vi "Initialize Sessions Impl.vi"(6 "initialize and close session behavior":T1, 7 "require single session":bool, 8 "error in":errorcluster, 10 "instrument":refnum<class "ISession Factory.lvclass">, 11 "session reservation in":refnum<class "Session Reservation.lvclass">) -> (0 "error out":errorcluster, 1 "channel lists":string[](array[string]), 2 "sessions":variant[](array[variant]), 3 "session reservation out":refnum<class "Session Reservation.lvclass">, 4 "location unique id":u64, 5 "retry":bool)   [LabVIEW 2020, in "Measurement Plugin Session Management V1.lvlib" / "Session Reservation.lvclass"]
uses:
  Session Reservation.lvclass
  Sessions/Instrument Sessions/ISession Factory/ISession Factory.lvclass
  Initialize and Close Session Behavior.ctl
  Session Reservation.lvclass/Session Reservation.ctl
  Sessions/Instrument Sessions/ISession Factory/Session Initialization Parameters.ctl
  Measurement Plugin Measurement Server/Helpers/Error Strings Global Internal.vi
  Connection Map/Connection Map.lvclass
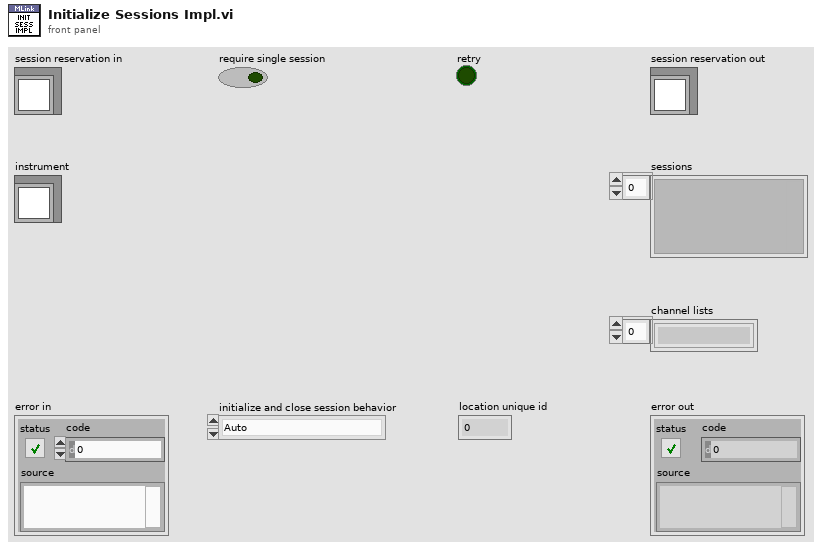
[diagram p1: front panel]
types:
  T1 = typedef "Measurement Plugin Session Management V1.lvlib/Session Reservation.lvclass/Initialize and Close Session Behavior.ctl" = enum16{"Auto", "Initialize and Close", "Attach and Detach", "Initialize and Detach", "Attach and Close"}
  T2 = typedef "Instrument Sessions.lvlib/ISession Factory.lvclass/Session Initialization Parameters.ctl" = cluster{"resource name":string, "session name":string}
  T3 = typedef "Measurement Plugin Session Management V1.lvlib/Session Reservation.lvclass/Data.ctl" = cluster{"session and driver infos":T4[], "pin or relay names":string[], "connection map":refnum<class "Connection Map.lvclass">, "pin map context":T9, "reservation observer":refnum<class "IReservation Observer.lvclass">, "dvr valid":bool, "group mappings":T10}
  T4 = typedef "Measurement Plugin Session Management V1.lvlib/Session Reservation.lvclass/Session and Driver Info.ctl" = cluster{"session info":T5, "session":variant, "session factory":refnum<class "ISession Factory.lvclass">, "initialize and close session behavior":T8}
  T5 = typedef "MeasurementLink Session Management Client.lvlib/ni_measurementlink_sessionmanagement_v1_SessionInformation.ctl" = cluster{"session":T6, "resource_name":string, "channel_list":string, "instrument_type_id":string, "session_exists":bool, "channel_mappings":T7[]}
  T6 = typedef "MeasurementLink Session Management Client.lvlib/nidevice_grpc_Session.ctl" = cluster{"name":string}
  T7 = typedef "MeasurementLink Session Management Client.lvlib/ni_measurementlink_sessionmanagement_v1_ChannelMapping.ctl" = cluster{"pin_or_relay_name":string, "site":i32, "channel":string, "multiplexer_resource_name":string, "multiplexer_route":string}
  T8 = typedef "Instrument Sessions.lvlib/ISession Factory.lvclass/Initialize and Close Session Behavior.ctl" = enum16{"Initialize and Close", "Attach and Detach", "Initialize and Detach", "Attach and Close"}
  T9 = typedef "MeasurementLink Session Management Client.lvlib/ni_measurementlink_PinMapContext.ctl" = cluster{"pin_map_id":string, "sites":i32[]}
  T10 = typedef "Measurement Plugin Session Management V1.lvlib/Session Reservation.lvclass/Group Mapping.ctl" = map{string, string[]}
  T11 = typedef "Instrument Sessions.lvlib/ISession Factory.lvclass/Remote Connection Options.ctl" = cluster{"session name":string, "address":string, "port":u32}
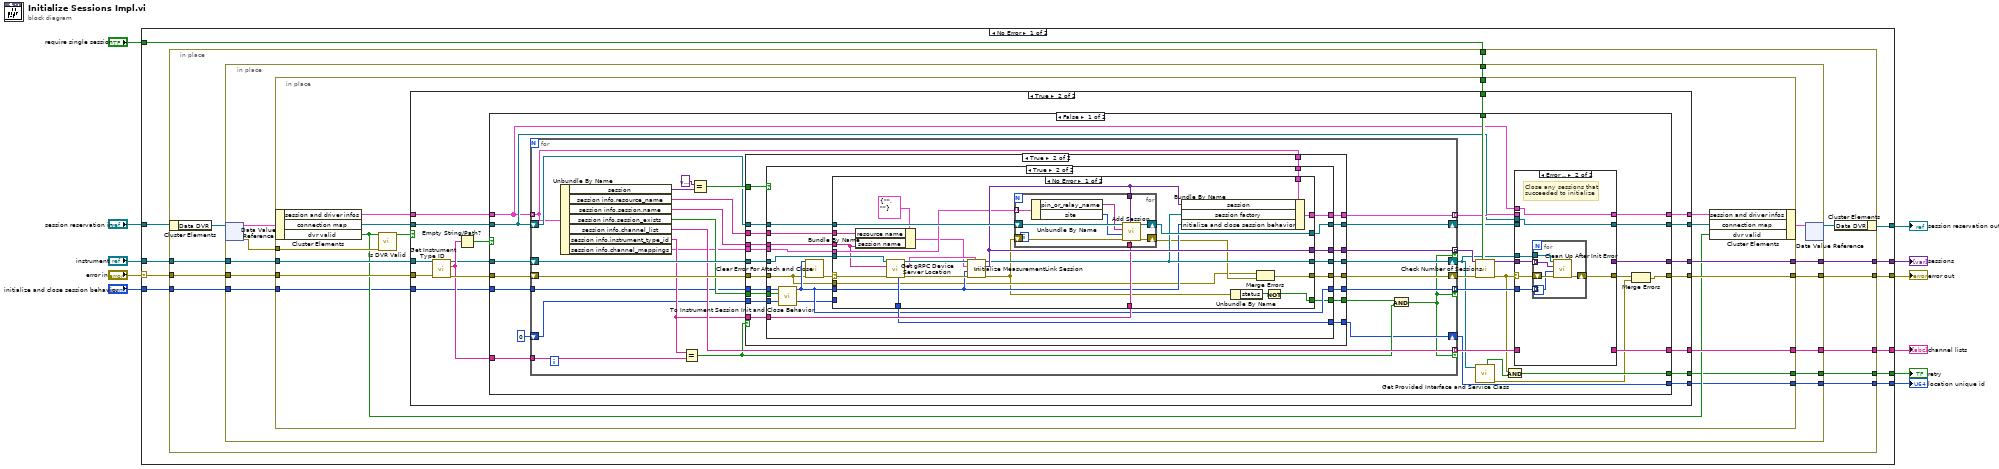
[diagram p0: block diagram]
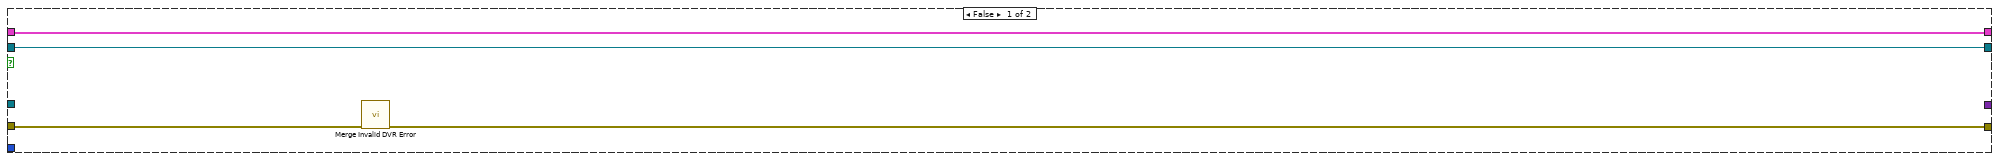
[diagram p2: hidden frame]
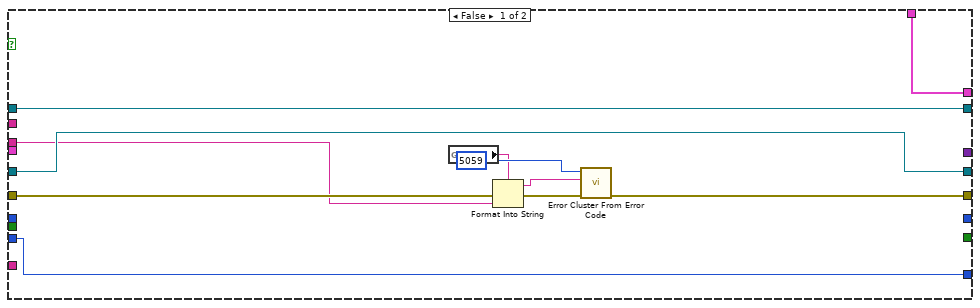
[diagram p5: hidden frame]
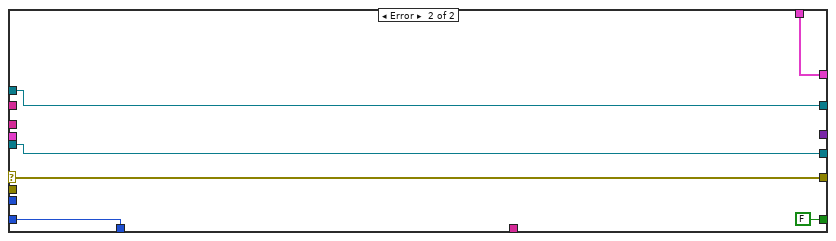
[diagram p6: hidden frame]
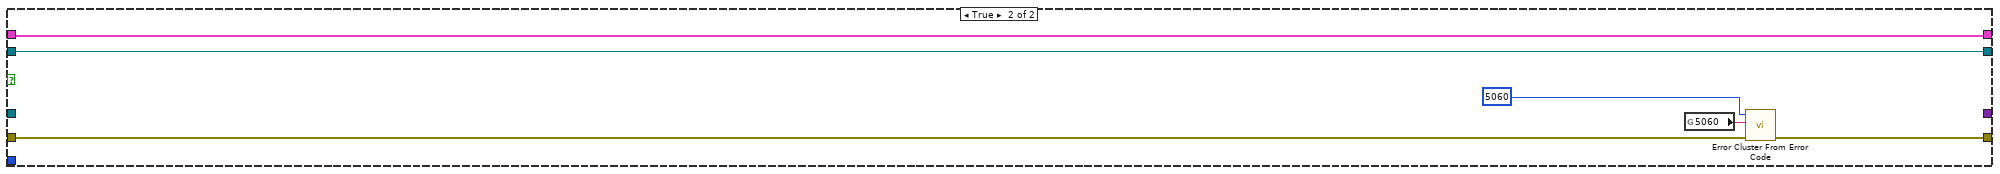
[diagram p7: hidden frame]
diagram:
  n1 = case shown="No Error" "error in" {
    selector: "error in" -> [w19 w256]
    tunnel: "session reservation in" -> [w16 w255]
    tunnel: "instrument" -> [w18 _]
    tunnel: [w22 _] -> w9
    tunnel: [w21 w256] -> w8
    tunnel: [w20 _] -> w7
    tunnel: [w15 w255] -> w4
    tunnel: "require single session" -> [w17 _]
    tunnel: "initialize and close session behavior" -> [w14 _]
    tunnel: [w13 _] -> w2
    tunnel: [w12 _] -> w1
    frame No Error {
      n2 = in-place {
        in-place-border: [w33] -> w22
        in-place-border: [w32] -> w21
        in-place-border: [w31] -> w20
        in-place-border: w19 -> [w30]
        in-place-border: w18 -> [w29]
        in-place-border: w17 -> [w28]
        in-place-border: w14 -> [w25]
        in-place-border: [w24] -> w13
        in-place-border: [w23] -> w12
        n3 = in-place-cluster #1(w16) -> ("Data DVR"=w27:refnum<data-value>)
        n4 = in-place {
          in-place-border: [w45] -> w33
          in-place-border: [w44] -> w32
          in-place-border: [w43] -> w31
          in-place-border: w30 -> [w42]
          in-place-border: w29 -> [w41]
          in-place-border: w28 -> [w40]
          in-place-border: w25 -> [w36]
          in-place-border: [w35] -> w24
          in-place-border: [w34] -> w23
          n5 = in-place-dvr #2(w27) -> (w39:T3, w38:errorcluster)
          n6 = in-place {
            in-place-border: [w61] -> w45
            in-place-border: [w60] -> w44
            in-place-border: [w59] -> w43
            in-place-border: w42 -> [w51]
            in-place-border: w41 -> [w50]
            in-place-border: w40 -> [w58]
            in-place-border: w38 -> [w54]
            in-place-border: w36 -> [w48]
            in-place-border: [w47] -> w35
            in-place-border: [w46] -> w34
            n7 = in-place-cluster #3(w39) -> ("session and driver infos"=w57:T4[], "connection map"=w56:refnum<class "Connection Map.lvclass">, "dvr valid"=w49:bool)
            n8 = call "Is DVR Valid.vi"("dvr error in"=w54, "dvr valid in"=w49) -> ("dvr valid out"=w53:bool)  [unwired: 9 in]
            n9 = case shown="True" w53 {
              tunnel: [_ w82] -> w61
              tunnel: [w62 w81] -> w60
              tunnel: [_ w80] -> w59
              tunnel: w58 -> [_ w79]
              tunnel: [w64 w78] -> w52
              tunnel: w57 -> [w64 w77]
              tunnel: w56 -> [w65 w76]
              tunnel: [w65 w75] -> w55
              tunnel: w51 -> [w63 w74]
              tunnel: w50 -> [_ w73]
              tunnel: w48 -> [_ w68]
              tunnel: [_ w67] -> w47
              tunnel: [_ w66] -> w46
              frame False {
                n10 = call "Merge Invalid DVR Error.vi"("error in"=w63) -> ("error out"=w62:errorcluster)  [unwired: 10 in]
              }
              frame True {
                n11 = call-dynamic "Get Instrument Type ID.vi"("error in"=w74, "session factory in"=w73) -> ("error out"=w72:errorcluster, "instrument type id"=w71:string, "session factory out"=w70:refnum<class "ISession Factory.lvclass">)  [unwired: 7 in]
                n12 = Empty String/Path?(string/path=w71) -> (empty?=w69:bool)
                n13 = case shown="False" w69 {
                  tunnel: w77 -> [w93 w254]
                  tunnel: [w109 _] -> w82
                  tunnel: [w85 w251] -> w81
                  tunnel: [w107 _] -> w80
                  tunnel: [w95 w254] -> w78
                  tunnel: w71 -> [w106 _]
                  tunnel: w70 -> [w105 _]
                  tunnel: w72 -> [w104 w250]
                  tunnel: w79 -> [w103 _]
                  tunnel: w76 -> [w96 w249]
                  tunnel: [w94 w249] -> w75
                  tunnel: w68 -> [w92 _]
                  tunnel: [w90 _] -> w67
                  tunnel: [w86 _] -> w66
                  frame False {
                    n14 = for {
                      tunnel: w93 -> [w137] mode=indexing
                      tunnel: [w151] -> w99 mode=indexing if=w129
                      shift-right: [w131] -> w100
                      shift-left: w104 -> [w147]
                      tunnel: [w145] -> w101 mode=indexing if=w129
                      tunnel: [w150] -> w102 mode=indexing
                      tunnel: w106 -> [w149]
                      shift-right: [w139] -> w89
                      shift-left: w105 -> [w148]
                      shift-right: [w136] -> w97
                      shift-left: w96 -> [w138]
                      tunnel: w92 -> [w133]
                      tunnel: [w132] -> w91 mode=indexing if=w129
                      shift-right: [w130] -> w90
                      shift-left: u64 0 ("location unique id") -> [w127]
                      n15 = Unbundle By Name(w137) -> ("session"=w144:variant, "session info.resource_name"=w146:string, "session info.session.name"=w152:string, "session info.session_exists"=w140:bool, "session info.channel_list"=w145:string, "session info.instrument_type_id"=w135:string, "session info.channel_mappings"=w134:T7[])
                      n16 = Equal?(x=w135, y=w149) -> (x = y?=w141:bool)
                      n17 = Equal?(x=variant, y=w144) -> (x = y?=w143:bool)
                      n18 = case shown="True" w141 {
                        tunnel: w152 -> [_ w177]
                        tunnel: [_ w173] -> w151
                        tunnel: w146 -> [_ w176]
                        tunnel: w140 -> [_ w175]
                        tunnel: [w156 w174] -> w131
                        tunnel: w137 -> [w157 w172]
                        tunnel: [w157 w171] -> w150
                        tunnel: w148 -> [w155 w170]
                        tunnel: w147 -> [w156 w169]
                        tunnel: w143 -> [_ w168]
                        tunnel: [w155 w167] -> w139
                        tunnel: w138 -> [w154 w166]
                        tunnel: [w154 w165] -> w136
                        tunnel: w135 -> [_ w164]
                        tunnel: w134 -> [_ w163]
                        tunnel: w133 -> [_ w162]
                        tunnel: [_ w161] -> w132
                        tunnel: [w153 w160] -> w130
                        tunnel: [_ w159] -> w128
                        tunnel: w127 -> [w153 w158]
                        frame False {
                        }
                        frame True {
                          n19 = case shown="True" w168 {
                            tunnel: w177 -> [w180 w196]
                            tunnel: w176 -> [_ w197]
                            tunnel: w175 -> [_ w198]
                            tunnel: [w187 w191] -> w174
                            tunnel: [_ w203] -> w173
                            tunnel: w172 -> [w186 w208]
                            tunnel: [w186 w207] -> w171
                            tunnel: w170 -> [w181 w206]
                            tunnel: w169 -> [w185 w192]
                            tunnel: [w181 w200] -> w167
                            tunnel: w166 -> [w179 w205]
                            tunnel: [w179 w204] -> w165
                            tunnel: w164 -> [_ w202]
                            tunnel: w163 -> [_ w201]
                            tunnel: w162 -> [_ w199]
                            tunnel: [_ w193] -> w161
                            tunnel: [w178 w195] -> w160
                            tunnel: [_ w190] -> w159
                            tunnel: w158 -> [w178 w189]
                            frame False {
                              n20 = global read "Error Strings Global Internal.vi" "5059"() -> (w182:string)
                              n21 = Format Into String(format string=w182, error in=w185, w180) -> (resulting string=w183:string, error out=w184:errorcluster)  [unwired: 1 in]
                              n22 = call <vilib>:"Error Cluster From Error Code.vi"("error in (no error)"=w184, "error message (\"\")"=w183, "error code (0)"=5059) -> ("error out"=w187:errorcluster)  [unwired: 6 in]
                            }
                            frame True {
                              n23 = call "To Instrument Session Init and Close Behavior.vi"("session exists"=w198, "initialize and close session behavior"=w199) -> ("instrument initialize and close session behavior"=w193:T8)  [unwired: 9 in]
                              n24 = call "Clear Error For Attach and Close.vi"("error in"=w192, "instrument initialize and close session behavior"=w193) -> ("error out"=w194:errorcluster)  [unwired: 9 in]
                              n25 = case shown="No Error" w194 {
                                selector: w194 -> [w216 w245]
                                tunnel: w208 -> [w233 w248]
                                tunnel: [w232 w248] -> w207
                                tunnel: w206 -> [w231 w246]
                                tunnel: w205 -> [w228 w247]
                                tunnel: [w227 w247] -> w204
                                tunnel: [w226 _] -> w203
                                tunnel: w202 -> [w225 _]
                                tunnel: w201 -> [w224 _]
                                tunnel: [w223 w246] -> w200
                                tunnel: w197 -> [w221 _]
                                tunnel: w196 -> [w220 _]
                                tunnel: [w219 w243] -> w195
                                tunnel: w193 -> [w215 _]
                                tunnel: w192 -> [w213 _]
                                tunnel: [w212 w245] -> w191
                                tunnel: [w209 FALSE] -> w190
                                tunnel: w189 -> [_ w243]
                                frame No Error {
                                n26 = Bundle By Name(cluster=T2 {"resource name"="", "session name"=""} ("session initialization details"), "resource name"=w221, "session name"=w220) -> (w217:T2)
                                n27 = call "Get gRPC Device Server Location.vi"("error in"=w216, "session name"=w220, "instrument in"=w231) -> ("error out"=w229:errorcluster, "remote connection options"=w218:T11, "instrument out"=w230:refnum<class "ISession Factory.lvclass">, "location unique id"=w219:u64)  [unwired: 4 in, 1 out]
                                n28 = call-dynamic "Initialize MeasurementLink Session.vi"("remote connection options"=w218, "error in"=w229, "initialize and close session behavior"=w215, "session initialization parameters"=w217, "session factory in"=w230) -> ("error out"=w211:errorcluster, "session out"=w226:variant, "session factory out"=w223:refnum<class "ISession Factory.lvclass">)  [unwired: 4 in]
                                n29 = for {
                                tunnel: w226 -> [w238]
                                tunnel: w225 -> [w237]
                                shift-right: [w241] -> w227
                                shift-left: w228 -> [w242]
                                shift-right: [w239] -> w214
                                shift-left: w211 -> [w240]
                                tunnel: w224 -> [w236] mode=indexing
                                n30 = Unbundle By Name(w236) -> ("pin_or_relay_name"=w235:string, "site"=w234:i32)
                                n31 = call "Add Session.vi"("instrument type id"=w237, "session to add"=w238, "error in"=w240, "site"=w234, "pin or relay name"=w235, "connection map in"=w242) -> ("error out"=w239:errorcluster, "connection map out"=w241:refnum<class "Connection Map.lvclass">)  [unwired: 4 in]
                                }
                                n32 = Bundle By Name(cluster=w233, "session"=w226, "session factory"=w223, "initialize and close session behavior"=w215) -> (w232:T4)
                                n33 = Unbundle By Name(w211) -> ("status"=w210:bool)
                                n34 = Merge Errors(w213, w214) -> (w212:errorcluster)
                                n35 = Not(x=w210) -> (.not. x?=w209:bool)
                                }
                                frame Error {
                                }
                              }
                            }
                          }
                        }
                      }
                      n36 = And(x=w128, y=w141) -> (x .and. y?=w129:bool)
                    }
                    n37 = call "Check Number of Sessions.vi"("require single session"=w103, "error in"=w100, "sessions in"=w99) -> ("error out"=w87:errorcluster, "sessions out"=w98:variant[])  [unwired: 7 in]
                    n38 = call "Get Provided Interface and Service Class.vi"("instrument in"=w89) -> ("error out"=w84:errorcluster, "using device service"=w88:bool)  [unwired: 6 in, 3 out]
                    n39 = And(x=w87, y=w88) -> (x .and. y?=w86:bool)
                    n40 = case shown="Error .." w87 {
                      selector: w87 -> [w114 w117]
                      tunnel: [w114 w120] -> w108
                      tunnel: w98 -> [w113 w118]
                      tunnel: [w113 _] -> w109
                      tunnel: w102 -> [w112 _]
                      tunnel: [w112 w121] -> w95
                      tunnel: w101 -> [w111 _]
                      tunnel: [w111 _] -> w107
                      tunnel: w93 -> [_ w121]
                      tunnel: w89 -> [_ w119]
                      tunnel: w97 -> [w110 _]
                      tunnel: [w110 w116] -> w94
                      tunnel: w96 -> [_ w116]
                      tunnel: w91 -> [_ w115]
                      frame No Error {
                      }
                      frame Error {
                        # "Close any sessions that \nsucceeded to initialize"
                        n41 = for {
                          tunnel: w119 -> [w125]
                          tunnel: w118 -> [w124] mode=indexing
                          shift-right: [w126] -> w120
                          shift-left: w117 -> [w123]
                          tunnel: w115 -> [w122] mode=indexing
                          n42 = call-dynamic "Clean Up After Init Error.vi"("error in"=w123, "initialize and close session behavior"=w122, "session in"=w124, "session factory in"=w125) -> ("error out"=w126:errorcluster)  [unwired: 7 in]
                        }
                      }
                    }
                    n43 = Merge Errors(w108, w84) -> (w85:errorcluster)
                  }
                  frame True {
                    n44 = global read "Error Strings Global Internal.vi" "5060"() -> (w252:string)
                    n45 = call <vilib>:"Error Cluster From Error Code.vi"("error in (no error)"=w250, "error message (\"\")"=w252, "error code (0)"=5060) -> ("error out"=w251:errorcluster)  [unwired: 6 in]
                  }
                }
              }
            }
            n46 = in-place-cluster #3("session and driver infos"=w52, "connection map"=w55, "dvr valid"=w49) -> (w37:T3)
          }
          n47 = in-place-dvr #2(w37) -> (w26:refnum<data-value>)  [unwired: 1 out]
        }
        n48 = in-place-cluster #1("Data DVR"=w26) -> (w15:refnum<class "Session Reservation.lvclass">)
      }
    }
    frame Error {
    }
  }
  "error out" <- w8
  "sessions" <- w9
  "channel lists" <- w7
  "session reservation out" <- w4
  "retry" <- w1
  "location unique id" <- w2
